vi "Get State.vi"(8 "error in (no error)":errorcluster, 11 "DAQmx Digitizer in":refnum<class "DAQmx Digitizer.lvclass">) -> (0 "error out":errorcluster, 1 "Data ready":bool, 2 "Armed":bool, 3 "DAQmx Digitizer out":refnum<class "DAQmx Digitizer.lvclass">, 4 "Availiable Samples":u32, 5 "Finished":bool)   [LabVIEW 2015, in "DAQmx Digitizer.lvclass"]
uses:
  DAQmx Digitizer.lvclass
  DAQmx Digitizer.lvclass/DAQmx Digitizer.ctl
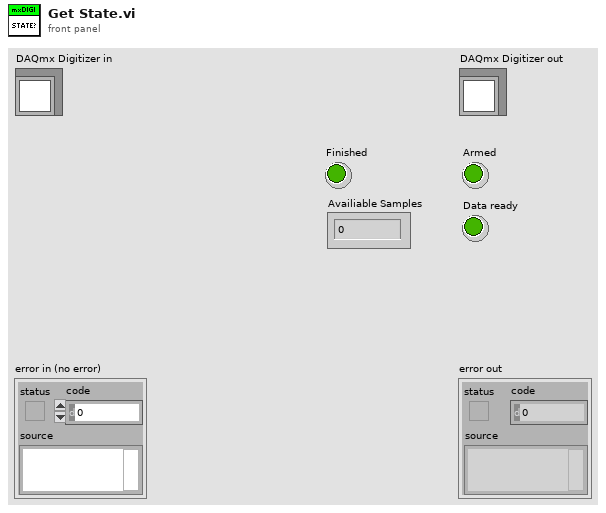
[diagram p1: front panel]
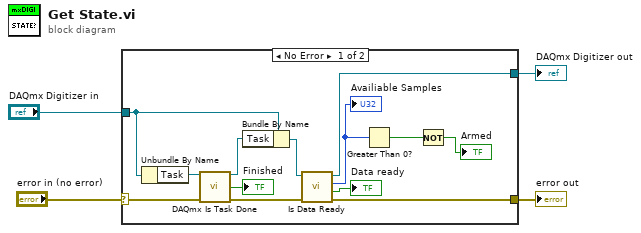
[diagram p0: block diagram]
diagram:
  n1 = case shown="No Error" "error in (no error)" {
    selector: "error in (no error)" -> [w14 w19]
    tunnel: [w6 w19] -> w3
    tunnel: [w10 w18] -> w1
    tunnel: "DAQmx Digitizer in" -> [w16 w18]
    frame No Error {
      n2 = Unbundle By Name(w16) -> ("Task"=w15:refnum<k21>)
      n3 = call <vilib>:"DAQmx Is Task Done.vi"("task/channels in"=w15, "error in"=w14) -> ("task out"=w13:refnum<k21>, "task done?"=→"Finished":bool, "error out"=w7:errorcluster)  [unwired: 11 out]
      n4 = Bundle By Name(cluster=w16, "Task"=w13) -> (w9:refnum<class "DAQmx Digitizer.lvclass">)
      n5 = call-dynamic "Is Data Ready.vi"("error in (no error)"=w7, "DAQmx Digitizer in"=w9) -> ("error out"=w6:errorcluster, "Data ready"=→"Data ready":bool, "Availiable Samples"=w8:u32, "DAQmx Digitizer out"=w10:refnum<class "DAQmx Digitizer.lvclass">)  [unwired: 6 in]
      "Availiable Samples" <- w8
      n6 = Greater Than 0?(x=w8) -> (x > 0?=w17:bool)
      n7 = Not(x=w17) -> (.not. x?=→"Armed":bool)
    }
    frame Error {
    }
  }
  "error out" <- w3
  "DAQmx Digitizer out" <- w1
